vi "LoadDataFromCloud.vi"(10 "FileName":string, 11 "CloudAddress":string) -> (1 "DataReadFromCloud(json)":string)   [LabVIEW 2017]
uses:
  <vilib>/httpClient/LabVIEWHTTPClient.lvlib
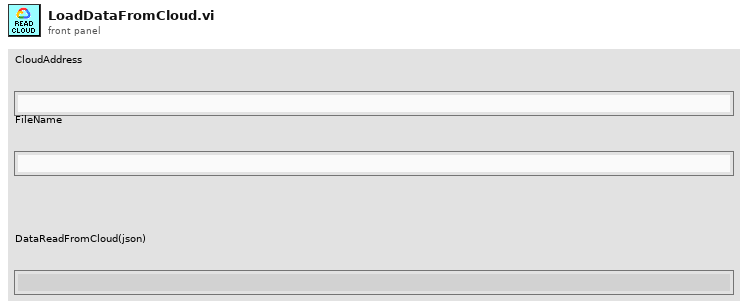
[diagram p1: front panel]
types:
  T1 = typedef "LabVIEWHTTPClient.lvlib/ClientHandle.ctl" = refnum<k1>
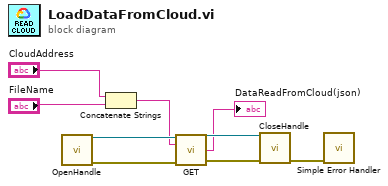
[diagram p0: block diagram]
diagram:
  n1 = call <vilib>:"OpenHandle.vi"() -> ("client handle out"=w9:T1, "error out"=w8:errorcluster)  [unwired: 14 in]
  n2 = Concatenate Strings("CloudAddress", "FileName") -> (w7:string)
  n3 = call <vilib>:"GET.vi"("client handle"=w9, "url"=w7, "error in (no error)"=w8) -> ("client handle out"=w4:T1, "body"=→"DataReadFromCloud(json)":string, "error out"=w3:errorcluster)  [unwired: 9 in, 1 out]
  n4 = call <vilib>:"CloseHandle.vi"("client handle"=w4, "error in (no error)"=w3) -> ("error out"=w2:errorcluster)  [unwired: 13 in]
  n5 = call <vilib>:"Simple Error Handler.vi"("error in (no error)"=w2) -> ()  [unwired: 4 in, 5 out]
